vi "LSR Terminal String.vi"() -> (3 "LSR Term":string="ÿÿÿÿÿÿÿÿÝÿÝÿÝÿÿ")   [LabVIEW 2015, in "LSR Instrument.lvlib"]
uses:
  LSR Instrument.lvlib
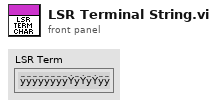
[diagram p1: front panel]
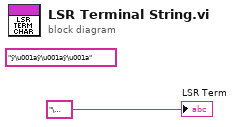
[diagram p0: block diagram]
diagram:
  (unwired) "ÿ\u001aÿ\u001aÿ\u001a" ("Termination Char(s)")
  "LSR Term" <- "\u0000" ("Termination Char(s)")
